vi "CRYProject Editor PIC Get Save Path.vi"(15 "error in":errorcluster) -> (4 "Path":path, 6 "Which Button?":T1(ring), 8 "Is Replace?":bool)   [LabVIEW 2013]
uses:
  CRYMainGlobal.vi
  CRYProject Editor Global.vi
panel:
  out "error out":errorcluster
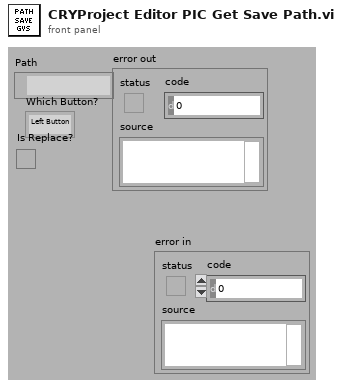
[diagram p1: front panel]
types:
  T1 = enum16{"Left Button", "Center Button", "Right Button", "Window Close"}
  T2 = typedef "CRYTS.ctl" = cluster{"No.TS":u16, "TS File Path":path, "TS Name":string, "EditStepName":string, "Steps":T3[], "New State":bool, "Change State":bool, "Flattened CurveLib Data":string, "Document Data":string, "EditStepNo":u16, "Operator Start File":string, "Sequence Type":string, "Sequence Language":string}
  T3 = typedef "CRYStep.ctl" = cluster{"No.VI":i32, "Category":string, "StepName":string, "Seq setup flattened":string, "Comment":string, "Steps config.":bool[], "Jump config":i32[], "Start":dbl, "Increment":dbl, "Name":string, "Unit":string, "Y data":u16, "Y prefix":string, "Y dB ref":dbl, "Y unit":string, "Repeat State Array":cluster{"Start":dbl, "Increment":dbl, "Count":i32, "Num":i32}[]}
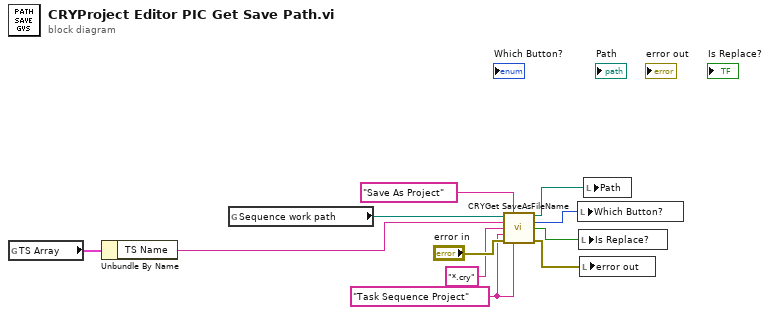
[diagram p0: block diagram]
diagram:
  w7 = "Task Sequence Project" ("pattern label")
  n1 = global read "CRYProject Editor Global.vi" "TS Array"() -> (w6:T2)
  n2 = Unbundle By Name(w6) -> ("TS Name"=w1:string)
  n3 = global read "CRYMainGlobal.vi" "Sequence work path"() -> (w11:path)
  n4 = call "CRYGet SaveAsFileName.vi"("Start path"=w11, "TitleName"="Save As Project" ("prompt"), "default name"=w1, "pattern (all files)"="*.cry" ("pattern label"), "pattern label"=w7, "error in"="error in", "Category Name"=w7) -> ("Path"=w5:path, "Which Button?"=w4:T1, "Is Replace?"=w3:bool, "error out"=w2:errorcluster)  [unwired: 4 in, 1 out]
  n5 = local write "Which Button?"(w4) -> ()
  n6 = local write "Is Replace?"(w3) -> ()
  n7 = local write "error out"(w2) -> ()
  n8 = local write "Path"(w5) -> ()
